vi "Init Object.vi"(10 "BG Color":u32(colorbox)) -> (3 "Dev Panel out":refnum<class "Dev Panel.lvclass">)   [LabVIEW 2021, in "Dev Panel.lvclass"]
uses:
  Dev Panel.lvclass
  Dev Panel.lvclass/Dev Panel.ctl
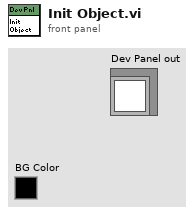
[diagram p1: front panel]
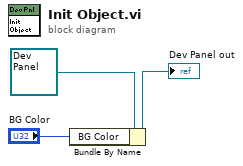
[diagram p0: block diagram]
diagram:
  n1 = Bundle By Name(cluster=refnum<class "Dev Panel.lvclass"> refnum ("Dev Panel in"), "BG Color"="BG Color") -> (→"Dev Panel out":refnum<class "Dev Panel.lvclass">)
